vi "Waveform Generator [Modified Express].vi"() -> ()   [LabVIEW 2017]
panel:
  out "error out":errorcluster
  in  "Waveform Parameters":T1={"Frequency"=50.0, "Amplitude"=5.0, "Shape"=enum."Sine"}
  out "XY Graph":cluster{"Displacement":dbl[], "Time":dbl[]}(graph)
  in  "stop":bool
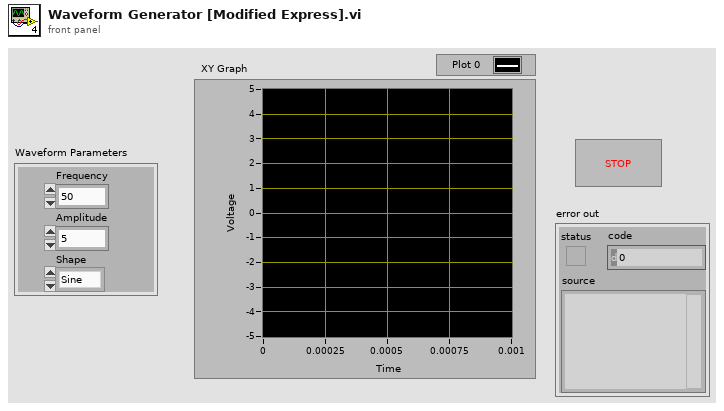
[diagram p1: front panel]
types:
  T1 = cluster{"Frequency":dbl, "Amplitude":dbl, "Shape":enum16{"Sine", "Cosine", "DC Level", "Square", "User-Defined"}}
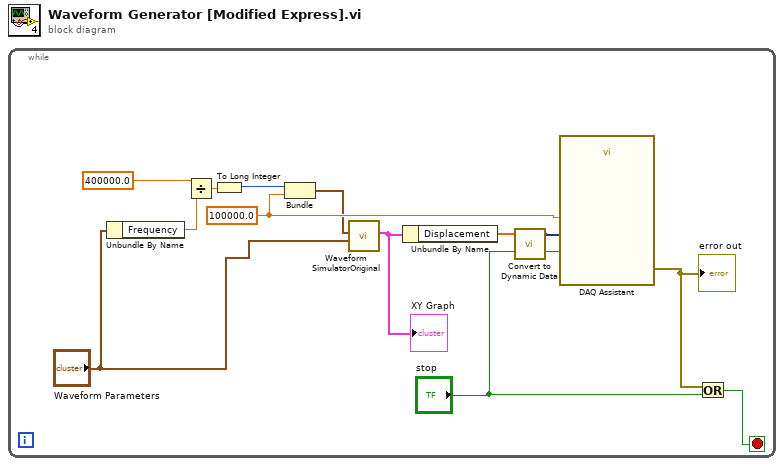
[diagram p0: block diagram]
diagram:
  n1 = while {
    stop <- w9 stop-if-true
    w2 = 100000.0
    n2 = Unbundle By Name("Waveform Parameters") -> ("Frequency"=w6:dbl)
    n3 = Divide(x=400000.0, y=w6) -> (x/y=w4:dbl)
    n4 = To Long Integer(number=w4) -> (32bit integer=w3:i32)
    n5 = Bundle(w3, w2) -> (w1:cluster{i32, dbl})  [unwired: 1 in]
    n6 = call "Waveform SimulatorOriginal.vi"("Waveform Parameters"="Waveform Parameters", "Digitizing Parameters"=w1) -> ("Waveform Output"=w8:cluster{"Time":dbl[], "Displacement":dbl[]})  [unwired: 9 in]
    "XY Graph" <- w8
    n7 = Unbundle By Name(w8) -> ("Displacement"=w13:dbl[])
    n8 = call "Convert to Dynamic Data"("Array"=w13) -> ("Dynamic Data Type"=w12:dynamicdata)  [unwired: 3 in]
    n9 = call "DAQ Assistant"("data"=w12, "rate"=w2, "stop (F)"="stop") -> ("error out"=w11:errorcluster)  [unwired: 14 in, 2 out]
    "error out" <- w11
    n10 = Or(x=w11, y="stop") -> (x .or. y?=w9:bool)
  }
